vi "Parse String with TDs__ogtk.vi"(8 "error in (no error)":errorcluster, 9 "offset (0)":i32, 10 "Data string":string, 11 "Type Descriptors":cluster{"Type Descriptor":T1}[](array[cluster])) -> (0 "error out":errorcluster, 1 "offset past parsing":i32, 2 "Array of VData":variant[](array[variant]))   [LabVIEW 2023, in "openg_variant.lvlib"]
doc: "Parses a flattened string with type descriptors to output an array of variant data."
uses:
  openg_variant.lvlib
  Type Descriptor__ogtk.ctl
panel:
  # "[OpenG VI Tags] ***Do Not Remove***"
  # "Parse String with TDs.vi\n\nParses a flattened string with type descriptors to output an array of variant da\n\nPlease visit http://www.OpenG.org to learn about the\nOpen Source LabVIEW software movement.\n\nNOTICE -- YOU MUST LEAVE THIS NOTICE IN PLACE.  PER THE TERMS OF THE LICENSE BELOW, YOU MAY SUBLICENSE THIS SOFTWARE \nIN ANY WAY THAT DOES NOT CONFLICT WITH THIS LICENSE.\n\n### BSD License (http://www.opensource.org/licenses/bsd-license.php) Begin ###\n \nCopyright (c) 2002, Jean-Pierre Drolet <drolet_jp@hotmail.com>\nCopyright (c) 2002-2006, Jim Kring <jim@jimkring.com>\n\nAll rights reserved.\n\nRedistribution and use in source and binary forms, with or without modification, are permitted provided that the following conditions are met:\n\n    * Redistributions of source code must retain the above copyright notice, this list of conditions and the following disclaimer.\n    * Redistributions in binary form must reproduce the above copyright notice, this list of conditions and the following disclaimer in the \n       documentation and/or other materials provided with the distribution.\n    * Neither the name of SciWare, James Kring, Inc., nor the names of its contributors may be used to endorse or promote products derived \n       from this software without specific prior written permission.\n\nTHIS SOFTWARE IS PROVIDED BY THE COPYRIGHT HOLDERS AND CONTRIBUTORS \"AS IS\" AND ANY EXPRESS OR IMPLIED WARRANTIES, \nINCLUDING, BUT NOT LIMITED TO, THE IMPLIED WARRANTIES OF MERCHANTABILITY AND FITNESS FOR A PARTICULAR PURPOSE ARE \nDISCLAIMED. IN NO EVENT SHALL THE COPYRIGHT OWNER OR CONTRIBUTORS BE LIABLE FOR ANY DIRECT, INDIRECT, INCIDENTAL,\n SPECIAL, EXEMPLARY, OR CONSEQUENTIAL DAMAGES (INCLUDING, BUT NOT LIMITED TO, PROCUREMENT OF SUBSTITUTE GOODS OR \nSERVICES; LOSS OF USE, DATA, OR PROFITS; OR BUSINESS INTERRUPTION) HOWEVER CAUSED AND ON ANY THEORY OF LIABILITY, \nWHETHER IN CONTRACT, STRICT LIABILITY, OR TORT (INCLUDING NEGLIGENCE OR OTHERWISE) ARISING IN ANY WAY OUT OF THE USE \nOF THIS SOFTWARE, EVEN IF ADVISED OF THE POSSIBILITY OF SUCH DAMAGE.\n\n### BSD License End ###"
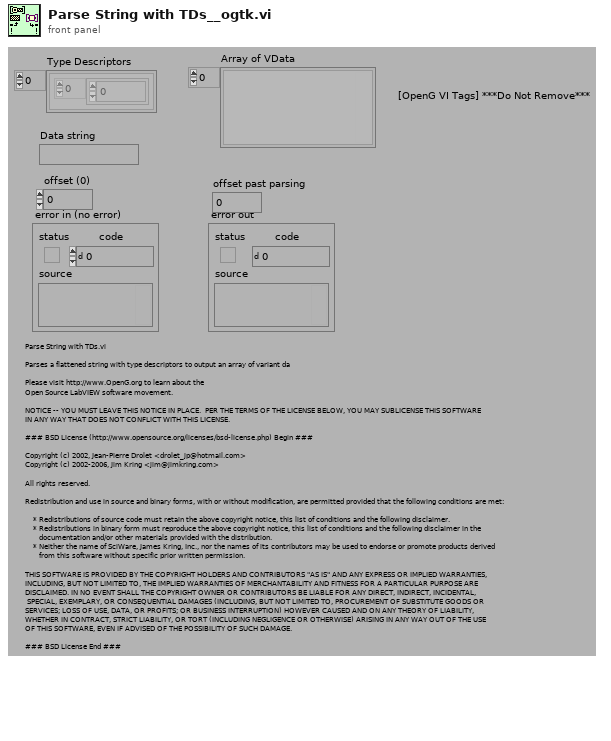
[diagram p1: front panel]
types:
  T1 = typedef "openg_variant.lvlib/Type Descriptor__ogtk.ctl" = i16[]
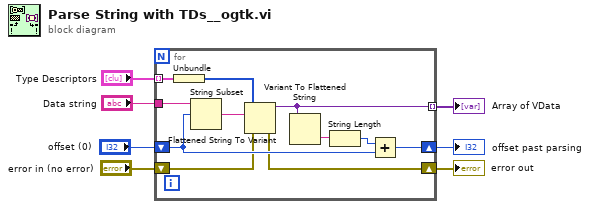
[diagram p0: block diagram]
diagram:
  n1 = for {
    tunnel: "Data string" -> [w15]
    tunnel: [w18] -> w4 mode=indexing
    shift-right: [w12] -> w1
    shift-left: "offset (0)" -> [w14]
    shift-right: [w10] -> w3
    shift-left: "error in (no error)" -> [w11]
    tunnel: "Type Descriptors" -> [w9] mode=indexing
    n2 = Unbundle(w9) -> ("Type Descriptor"=w8:T1)
    n3 = String Subset(string=w15, offset (0)=w14) -> (substring=w16:string)  [unwired: 1 in]
    n4 = Flattened String To Variant(4:w11, 6:w16, 7:w8) -> (0:w10:errorcluster, 3:w18:variant)
    n5 = Variant To Flattened String(Variant=w18) -> (data string=w17:string)  [unwired: 1 out]
    n6 = String Length(string=w17) -> (length=w13:i32)
    n7 = Add(x=w13, y=w14) -> (x+y=w12:i32)
  }
  "Array of VData" <- w4
  "error out" <- w3
  "offset past parsing" <- w1
